vi "Set_Audio_Device.vi"(8 "error in (no error)":errorcluster, 9 "AudioDevice":u16, 11 "speech_voice_refs":T1) -> (0 "error out":errorcluster, 1 "AudioDevice (out)":u16, 3 "speech_voice_refs (out)":T1)   [LabVIEW 8.6]
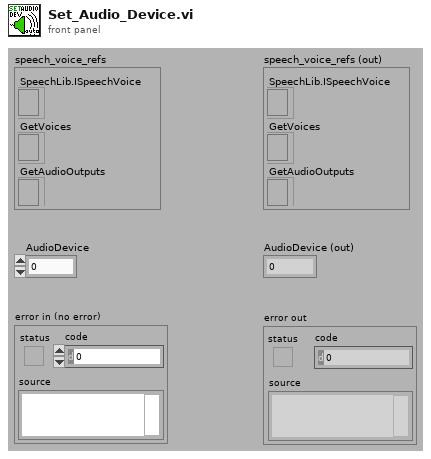
[diagram p1: front panel]
types:
  T1 = cluster{"SpeechLib.ISpeechVoice":refnum<k7>, "GetVoices":refnum<k7>, "GetAudioOutputs":refnum<k7>}
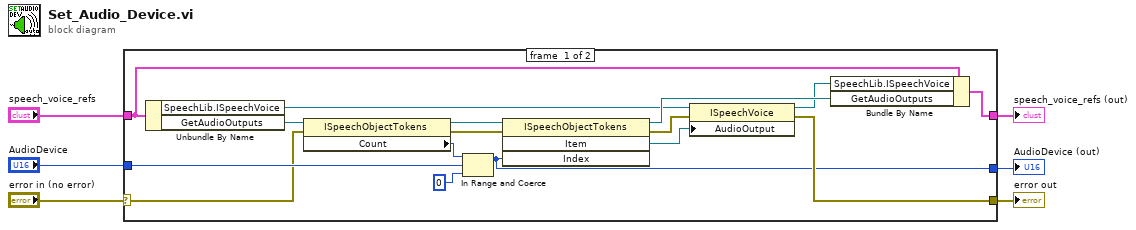
[diagram p0: block diagram]
diagram:
  n1 = case shown="No Error" "error in (no error)" {
    selector: "error in (no error)" -> [w9 w24]
    tunnel: "speech_voice_refs" -> [w22 w23]
    tunnel: [w21 w23] -> w5
    tunnel: [w10 w24] -> w4
    tunnel: "AudioDevice" -> [w17 _]
    tunnel: [w7 _] -> w1
    frame #0 {
      n2 = Unbundle By Name(w22) -> ("SpeechLib.ISpeechVoice"=w13:refnum<k7>, "GetAudioOutputs"=w20:refnum<k7>)
      n3 = property class="ISpeechObjectTokens"(reference=w20, error in=w9) -> (reference out=w16:refnum<k7>, error out=w12:errorcluster, "Count"=w19:i32)
      n4 = In Range and Coerce(upper limit=w19, x=w17, lower limit=0) -> (coerced(x)=w7:i32)  [unwired: 1 out]
      n5 = invoke class="ISpeechObjectTokens" method="Item"(reference=w16, error in=w12, "Index"=w7) -> (reference out=w15:refnum<k7>, error out=w11:errorcluster, "Item"=w14:refnum<k7>)  [unwired: 1 in, 1 out]
      n6 = property class="ISpeechVoice"(reference=w13, error in=w11, "AudioOutput"=w14) -> (reference out=w8:refnum<k7>, error out=w10:errorcluster)
      n7 = Bundle By Name(cluster=w22, "SpeechLib.ISpeechVoice"=w8, "GetAudioOutputs"=w15) -> (w21:T1)
    }
    frame #1 {
    }
  }
  "error out" <- w4
  "speech_voice_refs (out)" <- w5
  "AudioDevice (out)" <- w1
